vi "Auto Elevator Finger.vi"(7 "Elevator in Position":bool, 8 "Hold Low":bool, 9 "Idle Mode":T1, 10 "Has Trashcan":bool) -> (3 "Finger On?":bool)   [LabVIEW 2014]
uses:
  Common Code/Elevator Idle Mode.ctl
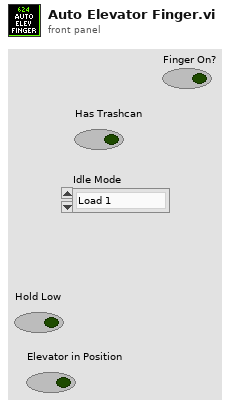
[diagram p1: front panel]
types:
  T1 = typedef "Elevator Idle Mode.ctl" = enum16{"Load 1", "Load 2", "Load 3", "Load Can", "Untip Can", "Step Load", "Drop Stack", "Raw Height"}
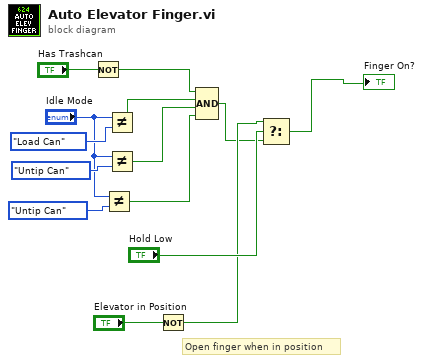
[diagram p0: block diagram]
diagram:
  # "Open finger when in position"
  n1 = Not(x="Has Trashcan") -> (.not. x?=w2:bool)
  n2 = Not Equal?(x="Idle Mode", y=Elevator_Idle_Mode."Untip Can") -> (x != y?=w5:bool)
  n3 = Not Equal?(x="Idle Mode", y=Elevator_Idle_Mode."Load Can") -> (x != y?=w3:bool)
  n4 = Not Equal?(x="Idle Mode", y=Elevator_Idle_Mode."Untip Can") -> (x != y?=w4:bool)
  n5 = Not(x="Elevator in Position") -> (.not. x?=w11:bool)
  n6 = Compound Arithmetic op=AND(w2, w3, w4, w5) -> (w1:bool)
  n7 = Select(t=w11, s="Hold Low", f=w1) -> (s? t:f=→"Finger On?":bool)
